vi "Sort filenames.vi"(11 "filenames":string[](array[string])) -> (3 "Sorted filenames":string[](array[string]))   [LabVIEW 2011]
panel:
  out "number":i32[](array[numeric])
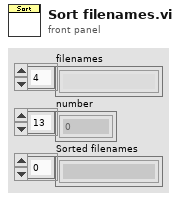
[diagram p1: front panel]
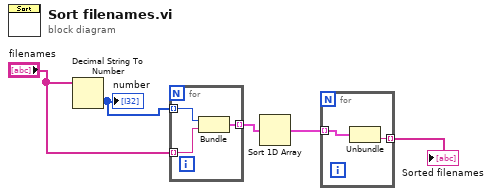
[diagram p0: block diagram]
diagram:
  n1 = Decimal String To Number(string="filenames") -> (number=w5:i32[])  [unwired: 2 in, 1 out]
  "number" <- w5
  n2 = for {
    tunnel: w5 -> [w8] mode=indexing
    tunnel: "filenames" -> [w7] mode=indexing
    tunnel: [w6] -> w3 mode=indexing
    n3 = Bundle(w8, w7) -> (w6:cluster{i32, string})  [unwired: 1 in]
  }
  n4 = Sort 1D Array(array=w3) -> (sorted array=w2:cluster{i32, string}[])
  n5 = for {
    tunnel: w2 -> [w10] mode=indexing
    tunnel: [w9] -> w1 mode=indexing
    n6 = Unbundle(w10) -> (w9:string)  [unwired: 1 out]
  }
  "Sorted filenames" <- w1
